vi "Close.vi"(8 "error in (no error)":errorcluster, 11 "DAQmx Base in":refnum<class "NI DAQmx Base.lvclass">) -> (0 "error out":errorcluster, 3 "DAQmx Base out":refnum<class "NI DAQmx Base.lvclass">)   [LabVIEW 2020, in "NI DAQmx.lvlib" / "NI DAQmx Base.lvclass"]
uses:
  NI DAQmx Base.lvclass
  NI DAQmx Base.lvclass/NI DAQmx Base.ctl
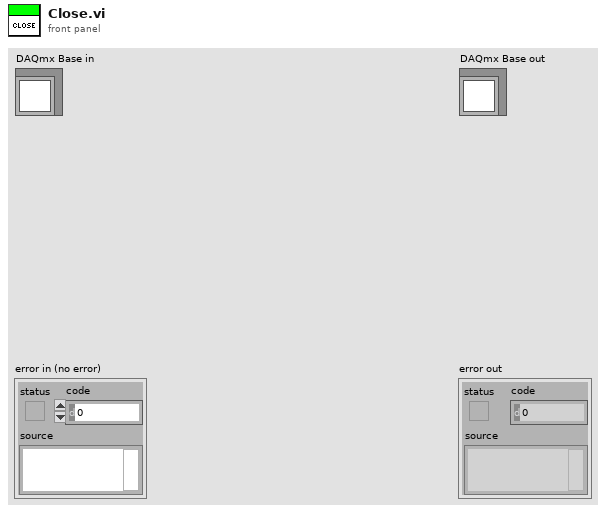
[diagram p1: front panel]
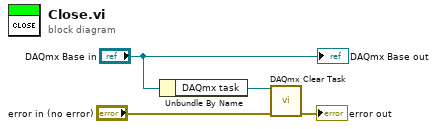
[diagram p0: block diagram]
diagram:
  n1 = Unbundle By Name("DAQmx Base in") -> ("DAQmx task"=w3:refnum<k21>)
  n2 = call <vilib>:"DAQmx Clear Task.vi"("task in"=w3, "error in"="error in (no error)") -> ("error out"=→"error out":errorcluster)  [unwired: 13 in]
  "DAQmx Base out" <- "DAQmx Base in"
